vi "RC_Generate_Test_Data.vi"(10 "Condition #":i32=1, 11 "Reward_Condition in":refnum<class "Reward_Condition.lvclass">) -> (3 "Reward_Condition out":refnum<class "Reward_Condition.lvclass">)   [LabVIEW 2018, in "Tracker.lvlib" / "Reward_Condition.lvclass"]
uses:
  Reward_Condition/Reward_Condition.lvclass
  Reward_SubCondition.lvclass
  Reward_Condition/Reward_Condition.lvclass/Reward_Condition.ctl
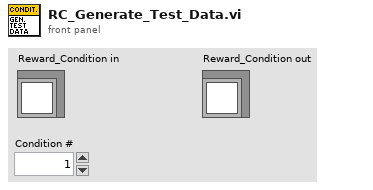
[diagram p1: front panel]
types:
  T1 = cluster{"Enabled":bool, "Type":enum16{"Angle to wall", "Speed", "Zone"}, "Comparison type":enum16{"Less", "Less or Equal", "Equal", "Greater or Equal", "Greater", "Not Equal"}, "Comparison value":dbl, "Validity check Enabled":bool, "Criteria to check":enum16{"Running bout, sec", "Running bout, m"}, "Has been True for, units":dbl}
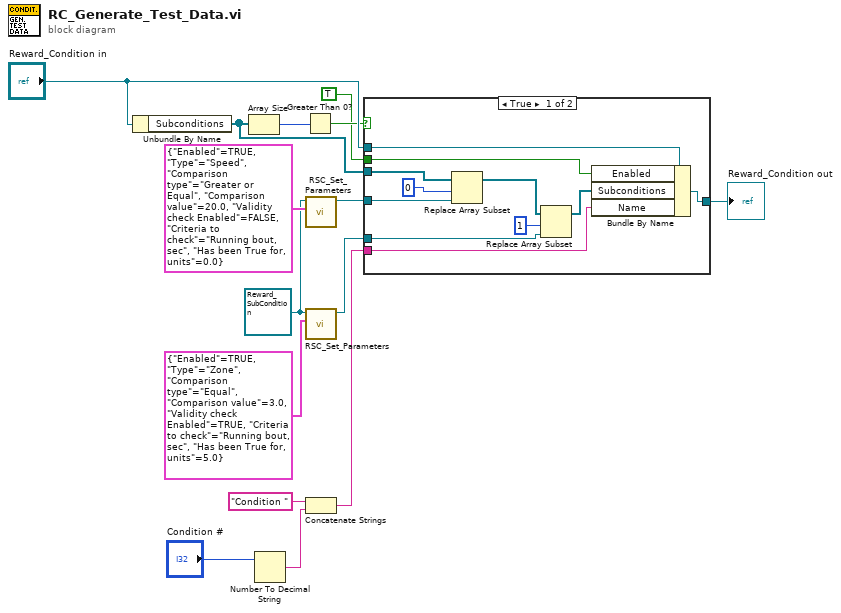
[diagram p0: block diagram]
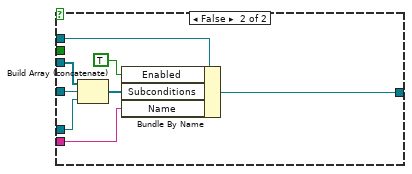
[diagram p2: hidden frame]
diagram:
  w3 = refnum<class "Reward_SubCondition.lvclass"> refnum ("new element/subarray")
  n1 = Unbundle By Name("Reward_Condition in") -> ("Subconditions"=w13:refnum<class "Reward_SubCondition.lvclass">[])
  n2 = Array Size(array=w13) -> (size(s)=w12:i32)
  n3 = Number To Decimal String(number="Condition #") -> (decimal integer string=w8:string)  [unwired: 1 in]
  n4 = Greater Than 0?(x=w12) -> (x > 0?=w11:bool)
  n5 = call "RSC_Set_Parameters.vi"("Data to update"=T1 {"Enabled"=TRUE, "Type"=enum."Speed", "Comparison type"=enum."Greater or Equal", "Comparison value"=20.0, "Validity check Enabled"=FALSE, "Criteria to check"=enum."Running bout, sec", "Has been True for, units"=0.0}, "Reward_SubCondition in"=w3) -> ("Reward_SubCondition out"=w1:refnum<class "Reward_SubCondition.lvclass">)  [unwired: 8 in, 1 out]
  n6 = call "RSC_Set_Parameters.vi"("Data to update"=T1 {"Enabled"=TRUE, "Type"=enum."Zone", "Comparison type"=enum."Equal", "Comparison value"=3.0, "Validity check Enabled"=TRUE, "Criteria to check"=enum."Running bout, sec", "Has been True for, units"=5.0}, "Reward_SubCondition in"=w3) -> ("Reward_SubCondition out"=w2:refnum<class "Reward_SubCondition.lvclass">)  [unwired: 8 in, 1 out]
  n7 = Concatenate Strings("Condition " ("string"), w8) -> (w6:string)
  n8 = case shown="True" w11 {
    tunnel: [w23 w34] -> w15
    tunnel: "Reward_Condition in" -> [w21 w32]
    tunnel: w13 -> [w20 w31]
    tunnel: w6 -> [w19 w29]
    tunnel: TRUE ("Enabled") -> [w18 _]
    tunnel: w2 -> [w17 w27]
    tunnel: w1 -> [w16 w28]
    frame True {
      n9 = Replace Array Subset(array=w20, new element=w16, index=0) -> (w24:refnum<class "Reward_SubCondition.lvclass">[])
      n10 = Replace Array Subset(array=w24, new element=w17, index=1) -> (w26:refnum<class "Reward_SubCondition.lvclass">[])
      n11 = Bundle By Name(cluster=w21, "Enabled"=w18, "Subconditions"=w26, "Name"=w19) -> (w23:refnum<class "Reward_Condition.lvclass">)
    }
    frame False {
      n12 = Build Array (concatenate)(w31, w28, w27) -> (w30:refnum<class "Reward_SubCondition.lvclass">[])
      n13 = Bundle By Name(cluster=w32, "Enabled"=TRUE, "Subconditions"=w30, "Name"=w29) -> (w34:refnum<class "Reward_Condition.lvclass">)
    }
  }
  "Reward_Condition out" <- w15
